vi "BRig_dataLC_Wrong_Block_l1.vi"() -> (2 "output_Wrong_Block":i32)   [LabVIEW 2014]
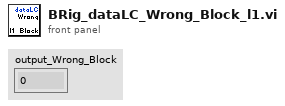
[diagram p1: front panel]
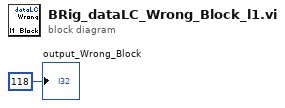
[diagram p0: block diagram]
diagram:
  "output_Wrong_Block" <- 118 ("output_iBlock")
